vi "NewIMAQImage.vi"(8 "error in (no error)":errorcluster, 10 "DeviceName":string, 11 "Photometrics Cam v2 in":refnum<class "CS250-CameraHardwareClass.lvclass">) -> (0 "error out":errorcluster, 3 "Photometrics Cam v2 out":refnum<class "CS250-CameraHardwareClass.lvclass">)   [LabVIEW 2013, in "CS250-CameraHardwareClass.lvclass"]
doc: "This VI creates and IMAQ image"
uses:
  CS250-CameraHardwareClass.lvclass
  CS250-CameraHardwareClass.lvclass/CS250-CameraHardwareClass.ctl
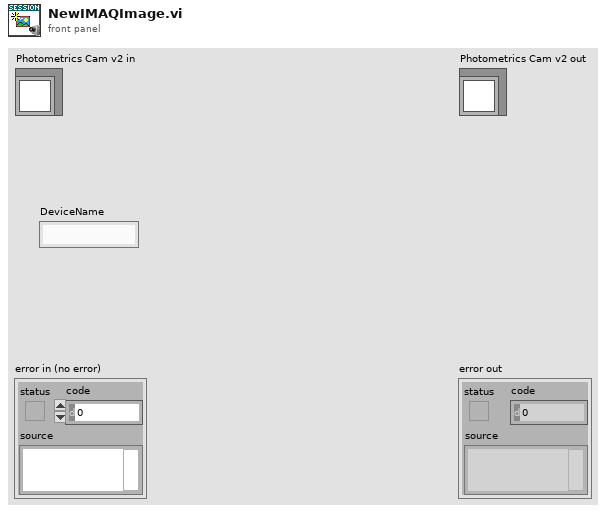
[diagram p1: front panel]
types:
  T1 = typedef "Image Type" = u32
  T2 = typedef "IMAQ Image.ctl" = refnum<image>
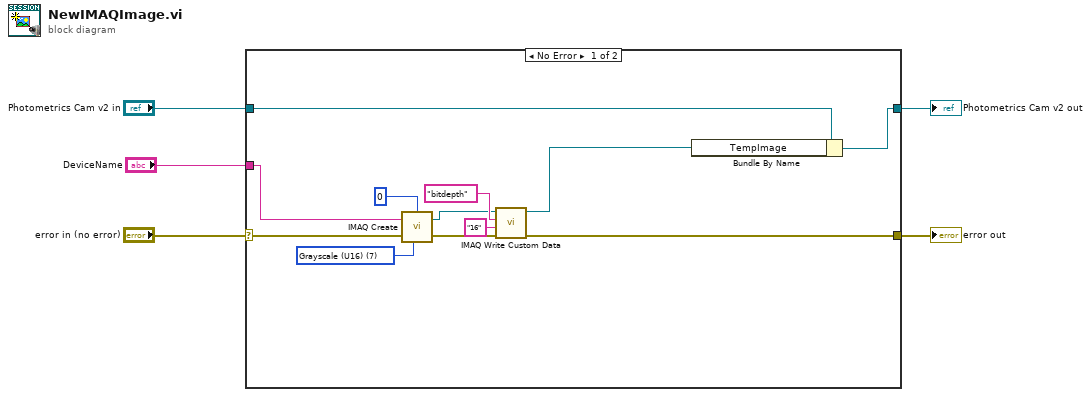
[diagram p0: block diagram]
diagram:
  n1 = case shown="No Error" "error in (no error)" {
    selector: "error in (no error)" -> [w15 w19]
    tunnel: [w6 w19] -> w4
    tunnel: [w14 w18] -> w2
    tunnel: "Photometrics Cam v2 in" -> [w8 w18]
    tunnel: "DeviceName" -> [w7 _]
    frame No Error {
      w16 = T1 7 items=["Grayscale (U8)", "Grayscale (I16)", "Grayscale (SGL)", "Complex (CSG)", "RGB (U32)", "HSL (U32)", "RGB (U64)", "Grayscale (U16)"] ("Image Type")
      n2 = call "IMAQ Create"("Border Size"=0, "Image Name"=w7, "Image Type"=w16, "error in (no error)"=w15) -> ("New Image"=w12:T2, "error out"=w11:errorcluster)  [unwired: 1 in]
      n3 = call "IMAQ Write Custom Data"("error in (no error)"=w11, "Custom Data In"="16", "Key"="bitdepth", "Image"=w12) -> ("error out"=w6:errorcluster, "Image Out"=w9:T2)  [unwired: 6 in]
      n4 = Bundle By Name(cluster=w8, "TempImage"=w9) -> (w14:refnum<class "CS250-CameraHardwareClass.lvclass">)
    }
    frame Error {
    }
  }
  "error out" <- w4
  "Photometrics Cam v2 out" <- w2
